vi "Close MeasurementLink Session.vi"(8 "error in":errorcluster, 9 "close session behavior":T1, 10 "session in":variant, 11 "session factory in":refnum<class "Session Factory.lvclass">) -> (0 "error out":errorcluster)   [LabVIEW 2021, in "Keysight 34461A DMM Instrument.lvlib" / "Session Factory.lvclass"]
uses:
  Session Factory.lvclass
  <vilib>/Plug-In SDKs/Sessions/Instrument/ISession Factory/ISession Factory.lvclass
  <instrlib>/Agilent 3446X Series/Public/Close.vi
  <instrlib>/Agilent 3446X Series/Agilent 3446X Series.lvlib
  <vilib>/Plug-In SDKs/Sessions/Instrument/ISession Factory/Initialize and Close Session Behavior.ctl
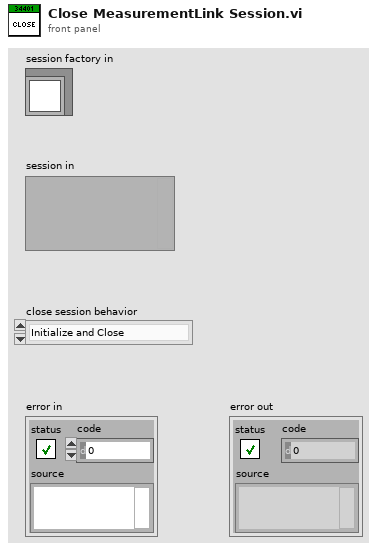
[diagram p1: front panel]
types:
  T1 = typedef "NI Session Management Instrument.lvlib/ISession Factory.lvclass/Initialize and Close Session Behavior.ctl" = enum16{"Initialize and Close", "Attach and Detach", "Initialize and Detach", "Attach and Close"}
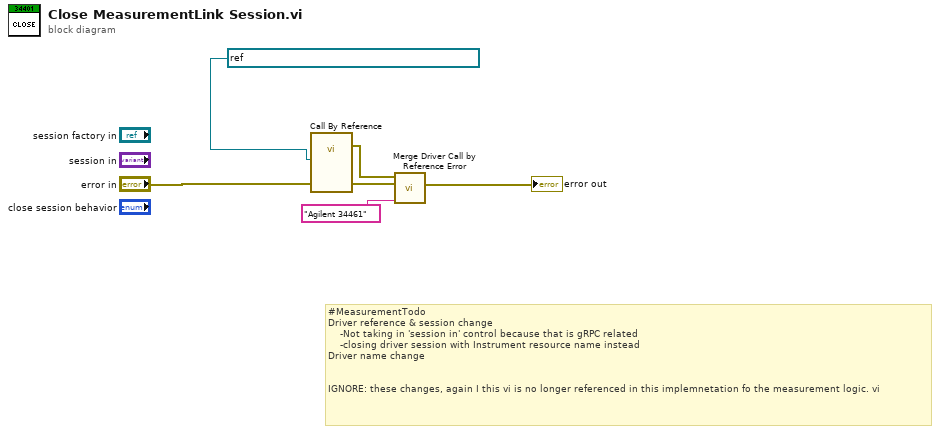
[diagram p0: block diagram]
diagram:
  # "#MeasurementTodo\nDriver reference & session change\n    -Not taking in 'session in' control because that is gRPC related\n    -closing driver session with Instrument resource name instead\nDriver name change\n\n\nIGNORE: these changes, again I this vi is no longer referenced in this implemnetation fo the measurement logic. vi"
  n1 = call-by-ref "?"("error in (no error)"="error in", "VISA resource name"=refnum<visa-resource-name> "USB0::0x2A8D::0x1301::MY53215615::INSTR" ("VISA resource name out")) -> (error out=w5:errorcluster, 0:"error out"=w4:errorcluster)  [unwired: 11 in, 1 out]
  n2 = call <vilib>:"Merge Driver Call by Reference Error.vi"("driver name"="Agilent 34461", "called vi error"=w4, "call by ref error"=w5) -> ("error out"=→"error out":errorcluster)  [unwired: 8 in]
